vi "K_S30c Terminal.vi"(4 "error in":errorcluster, 6 "request":u8[](array[numeric])) -> (0 "error out":errorcluster, 2 "response":u8[](array[numeric]))   [LabVIEW 2013]
uses:
  K_S30_VISA Global.vi
panel:
  in  "Case-Konstante\n(siehe Kontexthilfe)":bool
  out "msg and CRC":u8[](array[numeric])
  out "Echo":u8[](array[numeric])
  out "delited":u8[](array[numeric])
  # "Terminal for KELLER Transmitters Series3x \nVersion control:\nV1.0 15.11.2010  b.v. created\nV1.1 19.8.11 bv.MODBUS fct 1..16 & fct 20..23 added (for calibration only)\n\nConfigure ComPort: use K_S30 OpenComPort --> Global Variable\n\nsend a message with CRC16 checksum, receive the reponse\ncheck CRC16, and exceptions\n\nerrors:\n0: no error\n1,2,3,32: exceptions thrown by the device: see comm. protocol\n100: broadcast\n-2: wrong echo from the RS485 converter\n-4: timeout\n-5: CRC16 wrong\nothers thrown by VISA"
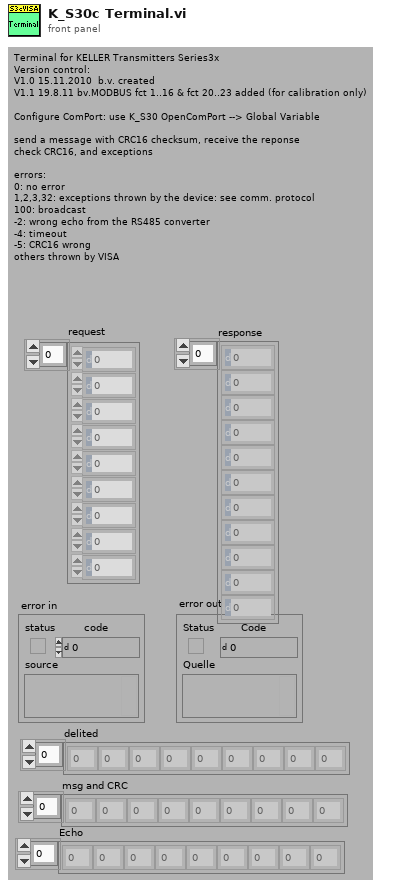
[diagram p1: front panel]
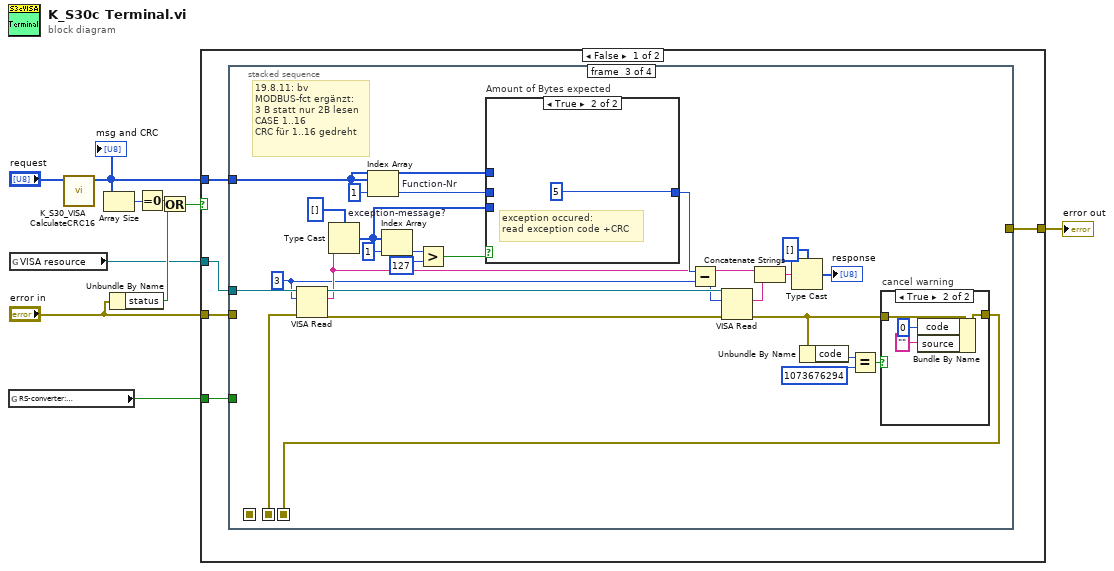
[diagram p0: block diagram]
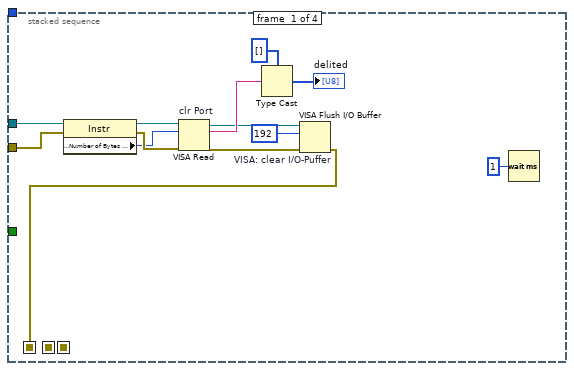
[diagram p2: hidden frame]
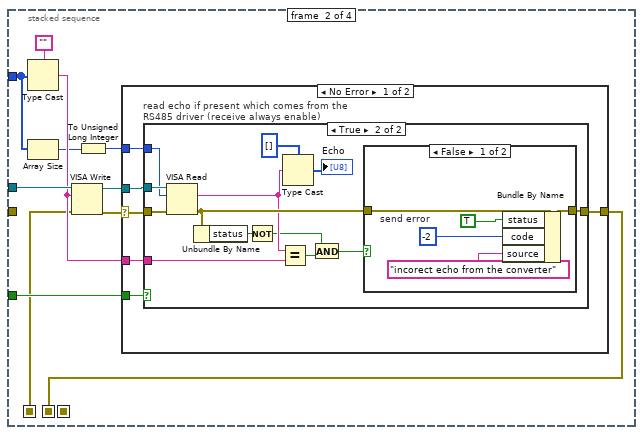
[diagram p3: hidden frame]
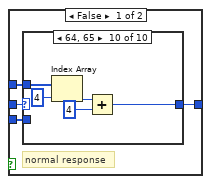
[diagram p8: hidden frame]
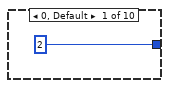
[diagram p9: hidden frame]
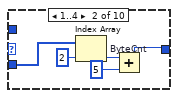
[diagram p10: hidden frame]
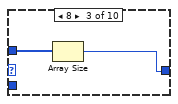
[diagram p11: hidden frame]
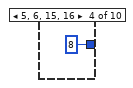
[diagram p12: hidden frame]
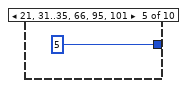
[diagram p13: hidden frame]
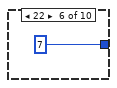
[diagram p14: hidden frame]
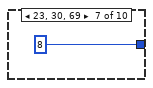
[diagram p15: hidden frame]
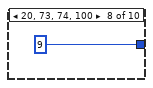
[diagram p16: hidden frame]
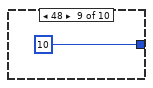
[diagram p17: hidden frame]
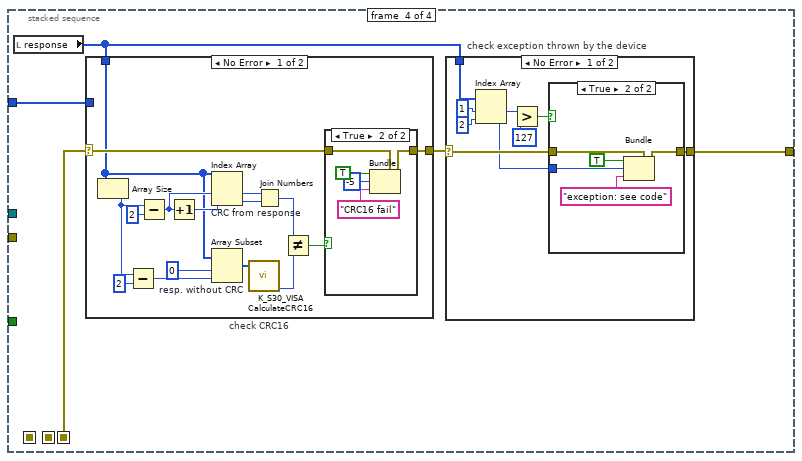
[diagram p18: hidden frame]
diagram:
  n1 = global read "K_S30_VISA Global.vi" "RS-converter:\necho"() -> (w2:bool)
  n2 = global read "K_S30_VISA Global.vi" "VISA resource"() -> (w1:refnum<visa-resource-name>)
  n3 = call "K_S30_VISA CalculateCRC16.vi"("msg without CRC"="request") -> ("msg and CRC"=w4:u8[])  [unwired: 3 in, 3 out]
  "msg and CRC" <- w4
  n4 = Array Size(array=w4) -> (size(s)=w5:i32)
  n5 = Unbundle By Name("error in") -> ("status"=w7:bool)
  n6 = Equal To 0?(x=w5) -> (x = 0?=w8:bool)
  n7 = Or(x=w8, y=w7) -> (x .or. y?=w6:bool)
  n8 = case shown="False" w6 {
    tunnel: w1 -> [w15 _]
    tunnel: "error in" -> [w14 w190]
    tunnel: w2 -> [w13 _]
    tunnel: w4 -> [w12 _]
    tunnel: [w11 w190] -> w3
    frame False {
      n9 = stacked-sequence {
        seq-local: [w18 _ _ _] -> [_ w30 _ _]
        seq-local: [_ w29 _ _] -> [_ _ w70 _]
        seq-local: [_ _ w71 _] -> [_ _ _ w123]
        tunnel: w15 -> [w16 w38 w91 _]
        tunnel: w14 -> [w24 _ _ _]
        tunnel: w13 -> [_ w37 _ _]
        tunnel: w12 -> [_ w34 w68 w122]
        tunnel: [_ _ _ w124] -> w11
        frame #0 {
          n10 = property class="Instr"(reference=w16, error in=w24) -> (reference out=w28:refnum<visa-resource-name>, error out=w27:errorcluster, "Serial Settings:Number of Bytes at Serial Port"=w26:u32)
          n11 = VISA Read "clr Port"(VISA resource name=w28, byte count=w26, error in (no error)=w27) -> (VISA resource name out=w20:refnum<visa-resource-name>, read buffer=w23:string, error out=w21:errorcluster)  [unwired: 1 out]
          n12 = Type Cast(type=u8[] [], x=w23) -> (*(type *) &x=→"delited":u8[])
          n13 = VISA Flush I/O Buffer "VISA: clear I/O-Puffer"(VISA resource name=w20, mask (16)=u16 192 ("Maskieren (16)"), error in (no error)=w21) -> (error out=w18:errorcluster)  [unwired: 1 out]
          n14 = Wait (ms)(milliseconds to wait=u32 1 ("ms Wartezeit")) -> ()  [unwired: 1 out]
        }
        frame #1 {
          n15 = Type Cast(type="", x=w34) -> (*(type *) &x=w35:string)
          n16 = Array Size(array=w34) -> (size(s)=w33:i32)
          n17 = VISA Write(VISA resource name=w38, write buffer=w35, error in (no error)=w30) -> (VISA resource name out=w39:refnum<visa-resource-name>, error out=w32:errorcluster)  [unwired: 1 out]
          n18 = To Unsigned Long Integer(number=w33) -> (unsigned 32bit integer=w31:u32)
          n19 = case shown="No Error" w32 {
            selector: w32 -> [w40 w66]
            tunnel: w39 -> [w45 _]
            tunnel: w37 -> [w44 _]
            tunnel: [w43 w66] -> w29
            tunnel: w35 -> [w42 _]
            tunnel: w31 -> [w41 _]
            frame No Error {
              n20 = case "read echo if present which comes from the RS485 driver (receive always enable)" shown="True" w44 {
                tunnel: w45 -> [_ w59]
                tunnel: w40 -> [w46 w58]
                tunnel: [w46 w53] -> w43
                tunnel: w42 -> [_ w57]
                tunnel: w41 -> [_ w47]
                frame False {
                }
                frame True {
                  n21 = VISA Read(VISA resource name=w59, byte count=w47, error in (no error)=w58) -> (read buffer=w52:string, error out=w56:errorcluster)  [unwired: 2 out]
                  n22 = Unbundle By Name(w56) -> ("status"=w55:bool)
                  n23 = Not(x=w55) -> (.not. x?=w49:bool)
                  n24 = Equal?(x=w52, y=w57) -> (x = y?=w48:bool)
                  n25 = Type Cast(type=u8[] [], x=w52) -> (*(type *) &x=→"Echo":u8[])
                  n26 = And(x=w49, y=w48) -> (x .and. y?=w54:bool)
                  n27 = case shown="False" w54 {
                    tunnel: w56 -> [w64 w65]
                    tunnel: [w63 w65] -> w53
                    frame False {
                      w60 = -2  # send error
                      n28 = Bundle By Name(cluster=w64, "status"=TRUE, "code"=w60, "source"="incorect echo from the converter") -> (w63:errorcluster)
                    }
                    frame True {
                    }
                  }
                }
              }
            }
            frame Error {
            }
          }
        }
        frame #2 {
          w69 = u32 3 ("Anzahl der Bytes (0)")
          # "19.8.11: bv\nMODBUS-fct ergänzt:\n3 B statt nur 2B lesen\nCASE 1..16\nCRC für 1..16 gedreht"
          n29 = VISA Read(VISA resource name=w91, byte count=w69, error in (no error)=w70) -> (VISA resource name out=w82:refnum<visa-resource-name>, read buffer=w79:string, error out=w83:errorcluster)  [unwired: 1 out]
          n30 = Type Cast(type=u8[] [], x=w79) -> (*(type *) &x=w67:u8[])
          n31 = Index Array "Function-Nr"(array=w68, index=1 ("Index")) -> (element=w85:u8)
          n32 = Index Array "exception-message?"(array=w67, index=1 ("Index")) -> (element=w89:u8)
          n33 = Greater?(x=w89, y=u8 127) -> (0:w87:bool)
          n34 = case "Amount of Bytes expected" shown="True" w87 {
            tunnel: w85 -> [w101 _]
            tunnel: [w100 u32 5] -> w84
            tunnel: w68 -> [w99 _]
            tunnel: w67 -> [w98 _]
            frame False {
              # "normal response"
              n35 = case shown="64, 65" w101 {
                tunnel: [u32 2 w103 w108 u32 8 u32 5 u32 7 u32 8 u32 9 u32 10 w116] -> w100
                tunnel: w99 -> [_ _ w109 _ _ _ _ _ _ w120]
                tunnel: w98 -> [_ w104 _ _ _ _ _ _ _ _]
                frame 0, Default {
                }
                frame 1..4 {
                  n36 = Index Array "ByteCnt"(array=w104, index=2 ("Index")) -> (element=w106:u8)
                  n37 = Add(x=w106, y=u8 5) -> (x+y=w103:u8)
                }
                frame 8 {
                  n38 = Array Size(array=w109) -> (size(s)=w108:i32)
                }
                frame 5, 6, 15, 16 {
                }
                frame 21, 31..35, 66, 95, 101 {
                }
                frame 22 {
                }
                frame 23, 30, 69 {
                }
                frame 20, 73, 74, 100 {
                }
                frame 48 {
                }
                frame 64, 65 {
                  n39 = Index Array(array=w120, index=4 ("Index")) -> (element=w118:u8)
                  n40 = Add(x=w118, y=u8 4) -> (x+y=w116:u8)
                }
              }
            }
            frame True {
              # "exception occured:\nread exception code +CRC"
            }
          }
          n41 = Subtract(x=w84, y=w69) -> (x-y=w81:u32)
          n42 = VISA Read(VISA resource name=w82, byte count=w81, error in (no error)=w83) -> (read buffer=w80:string, error out=w72:errorcluster)  [unwired: 2 out]
          n43 = Concatenate Strings(w79, w80) -> (w77:string)
          n44 = Type Cast(type=u8[] [], x=w77) -> (*(type *) &x=→"response":u8[])
          n45 = Unbundle By Name(w72) -> ("code"=w75:i32)
          n46 = Equal?(x=w75, y=1073676294 ("code")) -> (x = y?=w73:bool)
          n47 = case "cancel warning" shown="True" w73 {
            tunnel: w72 -> [w93 w97]
            tunnel: [w93 w94] -> w71
            frame False {
            }
            frame True {
              n48 = Bundle By Name(cluster=w97, "code"=0, "source"="") -> (w94:errorcluster)
            }
          }
        }
        frame #3 {
          n49 = local read "response"() -> (w125:u8[])
          n50 = case "check CRC16" shown="No Error" w123 {
            selector: w123 -> [w145 w169]
            tunnel: [w144 w168] -> w126
            tunnel: w125 -> [w143 _]
            tunnel: w122 -> [_ w165]
            frame No Error {
              n51 = Array Size(array=w143) -> (size(s)=w157:i32)
              n52 = Subtract(x=w157, y=2) -> (x-y=w155:i32)
              n53 = Subtract(x=w157, y=2) -> (x-y=w151:i32)
              n54 = Increment(x=w151) -> (x+1=w152:i32)
              n55 = Index Array "CRC from response"(array=w143, index #1=w151, index #2=w152) -> (element #1=w150:u8, element #2=w149:u8)
              n56 = Array Subset "resp. without CRC"(array=w143, index=0 ("Index"), length=w155) -> (w153:u8[])
              n57 = call "K_S30_VISA CalculateCRC16.vi"("msg without CRC"=w153) -> ("CRC16"=w147:u16)  [unwired: 3 in, 3 out]
              n58 = Join Numbers(hi=w150, lo=w149) -> ((hi.lo)=w148:u16)
              n59 = Not Equal?(x=w148, y=w147) -> (x != y?=w146:bool)
              n60 = case shown="True" w146 {
                tunnel: w145 -> [w159 w164]
                tunnel: [w159 w160] -> w144
                frame False {
                }
                frame True {
                  n61 = Bundle(cluster=w164, "status"=TRUE, "code"=-5, "source"="CRC16 fail") -> (w160:errorcluster)
                }
              }
            }
            frame Error {
              w171 = -1073807339  # timeout
              n62 = Unbundle By Name(w169) -> ("code"=w172:i32)
              n63 = Index Array(array=w165, index=0 ("Index")) -> (element=w166:u8)
              n64 = Equal?(x=w172, y=w171) -> (x = y?=w170:bool)
              n65 = case shown="True" w170 {
                tunnel: w169 -> [w173 w179]
                tunnel: [w173 w178] -> w168
                tunnel: w166 -> [_ w177]
                frame False {
                  # "other errors from VISA"
                  n66 = case shown="True" "Case-Konstante\n(siehe Kontexthilfe)" {
                    tunnel: w173 -> [_ w175]
                    frame False {
                    }
                    frame True {
                      n67 = call <vilib>:"Simple Error Handler.vi"("error in (no error)"=w175) -> ()  [unwired: 4 in, 5 out]
                    }
                  }
                }
                frame True {
                  n68 = Equal To 0?(x=w177) -> (x = 0?=w176:bool)
                  n69 = case "Braoadcast?" shown="True" w176 {
                    tunnel: w179 -> [w182 w186]
                    tunnel: [w181 w185] -> w178
                    frame False {
                      w180 = -4  # timeout
                      n70 = Bundle(cluster=w182, "status"=TRUE, "code"=w180, "source"="timeout") -> (w181:errorcluster)
                    }
                    frame True {
                      w187 = 100  # broadcast
                      n71 = Bundle(cluster=w186, "status"=TRUE, "code"=w187, "source"="broadcast") -> (w185:errorcluster)
                    }
                  }
                }
              }
            }
          }
          n72 = case "check exception thrown by the device" shown="No Error" w126 {
            selector: w126 -> [w130 w142]
            tunnel: [w129 w142] -> w124
            tunnel: w125 -> [w132 _]
            frame No Error {
              n73 = Index Array(array=w132, index #1=1 ("Index"), index #2=2 ("Index")) -> (element #1=w134:u8, element #2=w127:u8)
              n74 = Greater?(x=w134, y=u8 127) -> (0:w131:bool)
              n75 = case shown="True" w131 {
                tunnel: w130 -> [w136 w139]
                tunnel: [w136 w138] -> w129
                tunnel: w127 -> [_ w137]
                frame False {
                }
                frame True {
                  n76 = Bundle(cluster=w139, "status"=TRUE, "code"=w137, "source"="exception: see code") -> (w138:errorcluster)
                }
              }
            }
            frame Error {
            }
          }
        }
      }
    }
    frame True {
    }
  }
  "error out" <- w3
